vi "ClearError.vi"(9 "Error in":errorcluster) -> (1 "Error out":errorcluster)   [LabVIEW 2017, in "GPError.lvlib"]
doc: "Clears any error or warning on <B>Error in</B>, effectively returning an empty error cluster on <B>Error out</B>.\n\nThis VI is inlined.\n\nSteen Schmidt\nGPower\n16/12 2013"
uses:
  GPError.lvlib
panel:
  # "Copyright © 2013\nSteen Schmidt, GPower\nSee enclosed license file for terms and conditions"
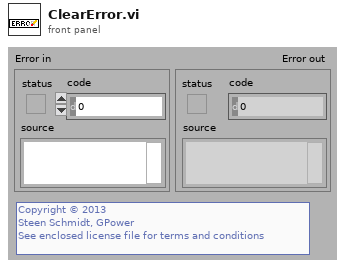
[diagram p1: front panel]
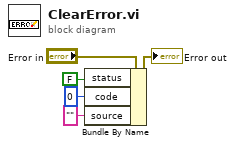
[diagram p0: block diagram]
diagram:
  n1 = Bundle By Name(cluster="Error in", "status"=FALSE, "code"=0, "source"="") -> (→"Error out":errorcluster)
